vi "manual_actions_write.vi"(8 "error in (no error)":errorcluster, 11 "manual_actions":variant) -> (0 "error out":errorcluster, 3 "actions_replaced":bool)   [LabVIEW 2015, in "lv-recipe-machine.lvlib"]
doc: "manual_actions_write.vi can be used to write one or more manual actions into the recipe_machine. Subsequent calls will aggregate all steps provided (no steps are deleted, but they can be replaced)."
uses:
  lv-recipe-machine.lvlib
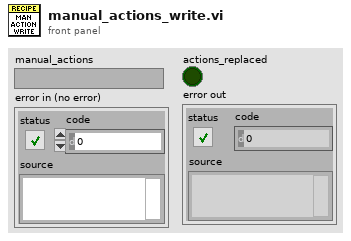
[diagram p1: front panel]
types:
  T1 = typedef "lv-recipe-machine.lvlib/references.ctl" = cluster{"semaphore":T2, "input_queue":refnum<queue>, "output_queue":refnum<queue>, "transition_queue":refnum<queue>, "data_dvr":refnum<data-value>, "stop_notifier":refnum<notifier>, "change_in_event":refnum<user-event>, "change_out_event":refnum<user-event>, "status_event":refnum<user-event>}
  T2 = typedef "Semaphore RefNum" = refnum<k1>
  T3 = typedef "lv-recipe-machine.lvlib/data.ctl" = cluster{"configuration":T4, "working":cluster{"recipe_data":T5}}
  T4 = typedef "lv-recipe-machine.lvlib/configuration.ctl" = cluster{"change_in_timeout_ms":i32}
  T5 = typedef "lv-recipe-machine.lvlib/recipe_data.ctl" = cluster{"mode":T6, "manual_state":T7, "automatic_state":T8, "previous_automatic_state":T8, "error":errorcluster, "timer []":T9[], "manual":cluster{"step_action":string, "data":variant, "actions":variant}, "automatic":cluster{"data":variant, "steps":variant, "criteria":variant, "transition":string, "index":i32, "step_launched":bool, "recipe []":T10[]}}
  T6 = typedef "lv-recipe-machine.lvlib/mode.ctl" = enum16{"<mode>", "manual", "automatic", "<null>"}
  T7 = typedef "lv-recipe-machine.lvlib/manual_state.ctl" = enum16{"<manual_state>", "failed", "action", "running", "idle", "<null>"}
  T8 = typedef "lv-recipe-machine.lvlib/automatic_state.ctl" = enum16{"<automatic_state>", "failed", "idle", "running", "paused", "stopped", "<null>"}
  T9 = typedef "lv-recipe-machine.lvlib/timer.ctl" = cluster{"elapsed_time":dbl, "previous_time":dbl}
  T10 = typedef "lv-recipe-machine.lvlib/recipe_step.ctl" = cluster{"step":string, "data":variant}
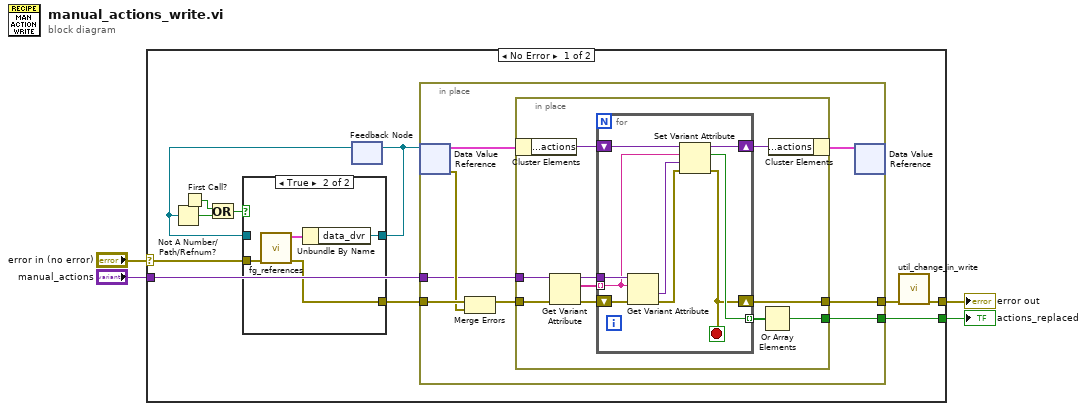
[diagram p0: block diagram]
diagram:
  n1 = case shown="No Error" "error in (no error)" {
    selector: "error in (no error)" -> [w5 w49]
    tunnel: [w15 w49] -> w3
    tunnel: "manual_actions" -> [w14 _]
    tunnel: [w12 _] -> w1
    frame No Error {
      n2 = First Call?() -> (First Call?: T/F=w10:bool)
      n3 = feedback #1() -> (w9:refnum<data-value>)  [unwired: 1 in]
      n4 = Not A Number/Path/Refnum?(number/path/refnum=w9) -> (NaN/Path/Refnum?=w11:bool)
      n5 = Or(x=w10, y=w11) -> (x .or. y?=w8:bool)
      n6 = case shown="True" w8 {
        tunnel: w5 -> [w16 w21]
        tunnel: [w16 w20] -> w6
        tunnel: [w17 w18] -> w7
        tunnel: w9 -> [w17 _]
        frame False {
        }
        frame True {
          n7 = call "fg_references.vi"("error in (no error)"=w21) -> ("error out"=w20:errorcluster, "references out"=w19:T1)  [unwired: 9 in]
          n8 = Unbundle By Name(w19) -> ("data_dvr"=w18:refnum<data-value>)
        }
      }
      n9 = feedback-in #1(w7) -> ()
      n10 = in-place {
        in-place-border: [w23] -> w13
        in-place-border: w6 -> [w29]
        in-place-border: w14 -> [w25]
        in-place-border: [w22] -> w12
        n11 = in-place-dvr #2(w7) -> (w27:T3, w28:errorcluster)
        n12 = Merge Errors(w29, w28) -> (w24:errorcluster)
        n13 = in-place {
          in-place-border: w25 -> [w37]
          in-place-border: w24 -> [w36]
          in-place-border: [w32] -> w23
          in-place-border: [w30] -> w22
          n14 = in-place-cluster #3(w27) -> ("working.recipe_data.manual.actions"=w39:variant)
          n15 = Get Variant Attribute(Variant=w37, error in=w36) -> (duplicate Variant=w35:variant, names=w34:string[], error out=w33:errorcluster)  [unwired: 2 in, 1 out]
          n16 = for {
            shift-right: [w47] -> w38
            shift-left: w39 -> [w48]
            tunnel: [w46] -> w31 mode=indexing
            tunnel: w35 -> [w44]
            tunnel: w34 -> [w40] mode=indexing
            shift-right: [w45] -> w32
            shift-left: w33 -> [w43]
            stop <- w45 stop-if-true
            n17 = Get Variant Attribute(Variant=w44, name=w40, error in=w43) -> (value=w41:variant, error out=w42:errorcluster)  [unwired: 1 in, 2 out]
            n18 = Set Variant Attribute(Variant=w48, name=w40, value=w41, error in=w42) -> (Variant out=w47:variant, replaced=w46:bool, error out=w45:errorcluster)
          }
          n19 = Or Array Elements(Boolean array=w31) -> (logical OR=w30:bool)
          n20 = in-place-cluster #3("working.recipe_data.manual.actions"=w38) -> (w26:T3)
        }
        n21 = in-place-dvr #2(w26) -> ()  [unwired: 2 out]
      }
      n22 = call "util_change_in_write.vi"("error in (no error)"=w13) -> ("error out"=w15:errorcluster)  [unwired: 10 in]
    }
    frame Error {
    }
  }
  "error out" <- w3
  "actions_replaced" <- w1
